vi "UDP Errors.vi"   [LabVIEW 2017, in "UDP.lvlib" / "UDP Transceiver.lvclass"]
uses:
  UDP Transceiver.lvclass
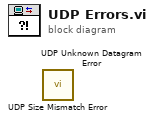
[diagram p0: block diagram]
diagram:
  n1 = call "UDP Size Mismatch Error.vi"() -> ()  [unwired: 10 in, 2 out]
  n2 = call "UDP Unknown Datagram Error.vi"() -> ()  [unwired: 10 in, 2 out]
